vi "Default Numeric Alarms (TT).vi"() -> (3 "Default Numeric Alarms":T1[](array[typedef]))   [LabVIEW 2018, in "Dynamic Shared Variables.lvlib"]
doc: "Create a numeric alarm configuration with some defaults."
uses:
  Dynamic Shared Variables.lvlib
  Tag VIs/Numeric Alarm Settings Cluster.ctl
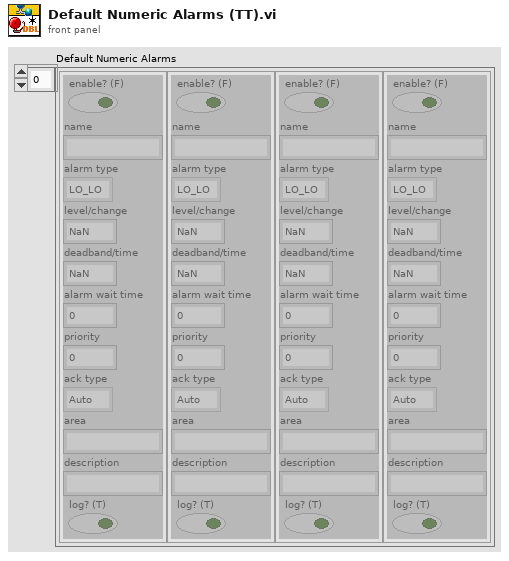
[diagram p1: front panel]
types:
  T1 = typedef "Numeric Alarm Settings Cluster.ctl" = cluster{"enable? (F)":bool, "name":string, "alarm type":enum16{"HI_HI", "HI", "LO", "LO_LO"}, "level/change":dbl, "deadband/time":dbl, "alarm wait time":dbl, "priority":u32, "ack type":enum16{"Auto", "User", "None", "Each Occurrence"}, "area":string, "description":string, "log? (T)":bool}
  T2 = cluster{"enable? (F)":bool, "name":string, "alarm type":enum16{"HI_HI", "HI", "LO", "LO_LO"}, "level/change":dbl, "deadband/time":dbl, "alarm wait time":dbl, "priority":u32, "ack type":enum16{"Auto", "User", "None", "Each Occurrence"}, "area":string, "description":string, "log? (T)":bool}[]
  T3 = cluster{"enable? (F)":bool, "name":string, "alarm type":enum16{"HI_HI", "HI", "LO", "LO_LO"}, "level/change":dbl, "deadband/time":dbl, "alarm wait time":dbl, "priority":u32, "ack type":enum16{"Auto", "User", "None", "Each Occurrence"}, "area":string, "description":string, "log? (T)":bool}
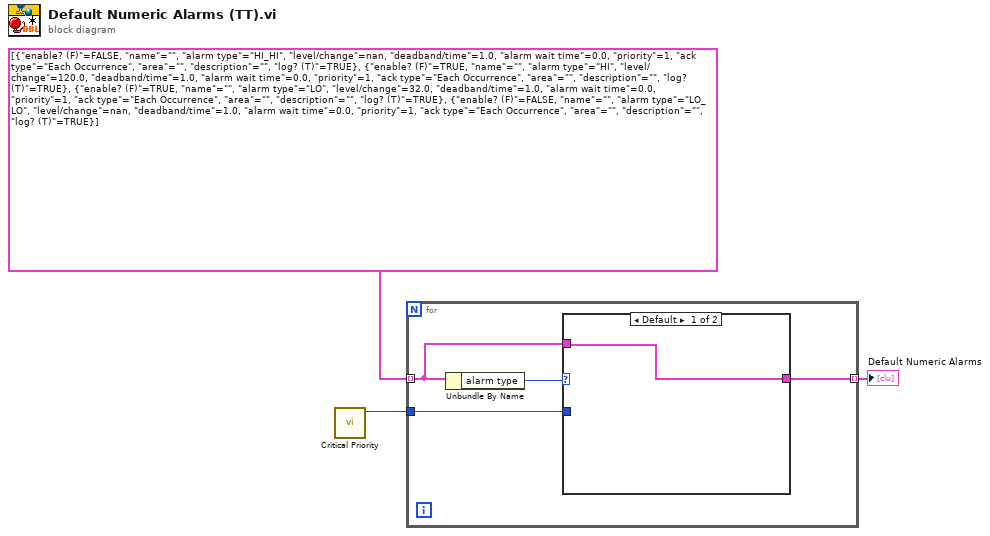
[diagram p0: block diagram]
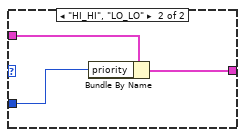
[diagram p2: hidden frame]
diagram:
  n1 = call "Critical Priority.vi"() -> ("critical priority"=w2:i32)  [unwired: 11 in]
  n2 = for {
    tunnel: T2 [{"enable? (F)"=FALSE, "name"="", "alarm type"=enum."HI_HI", "level/change"=nan, "deadband/time"=1.0, "alarm wait time"=0.0, "priority"=1, "ack type"=enum."Each Occurrence", "area"="", "description"="", "log? (T)"=TRUE}, {"enable? (F)"=TRUE, "name"="", "alarm type"=enum."HI", "level/change"=120.0, "deadband/time"=1.0, "alarm wait time"=0.0, "priority"=1, "ack type"=enum."Each Occurrence", "area"="", "description"="", "log? (T)"=TRUE}, {"enable? (F)"=TRUE, "name"="", "alarm type"=enum."LO", "level/change"=32.0, "deadband/time"=1.0, "alarm wait time"=0.0, "priority"=1, "ack type"=enum."Each Occurrence", "area"="", "description"="", "log? (T)"=TRUE}, {"enable? (F)"=FALSE, "name"="", "alarm type"=enum."LO_LO", "level/change"=nan, "deadband/time"=1.0, "alarm wait time"=0.0, "priority"=1, "ack type"=enum."Each Occurrence", "area"="", "description"="", "log? (T)"=TRUE}] -> [w7] mode=indexing
    tunnel: w2 -> [w5]
    tunnel: [w4] -> w1 mode=indexing
    n3 = Unbundle By Name(w7) -> ("alarm type"=w6:enum16{"HI_HI", "HI", "LO", "LO_LO"})
    n4 = case shown="Default" w6 {
      tunnel: w7 -> [w8 w11]
      tunnel: w5 -> [_ w10]
      tunnel: [w8 w9] -> w4
      frame Default {
      }
      frame "HI_HI", "LO_LO" {
        n5 = Bundle By Name(cluster=w11, "priority"=w10) -> (w9:T3)
      }
    }
  }
  "Default Numeric Alarms" <- w1
